vi "configureForCurrentOutput.vi"(8 "error in (no error)":errorcluster, 11 "AnalogOutput in":refnum<class "AnalogOutput.lvclass">) -> (0 "error out":errorcluster, 3 "AnalogOutput out":refnum<class "AnalogOutput.lvclass">)   [LabVIEW 2011, in "Hardware.lvlib" / "Channels.lvlib" / "AnalogOutput.lvclass"]
uses:
  AnalogOutput.lvclass
panel:
  in  "Output Properties":T1
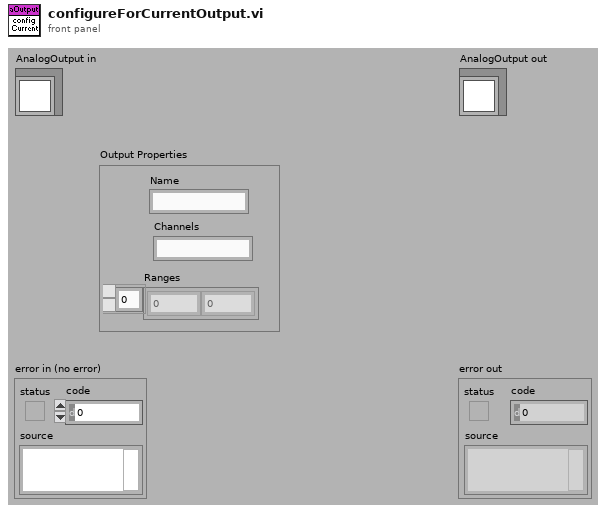
[diagram p1: front panel]
types:
  T1 = cluster{"Name":string, "Channels":string, "Ranges":dbl[]}
  T2 = cluster{"Configuration Type":cluster{"Differential":i16, "Pseudodifferential":i16, "RSE":dbl}, "Output Type":cluster{"Voltage":string, "Current":string, "Standard Function ":cluster{"Sine":string, "Square":string, "Triangle":string}}}
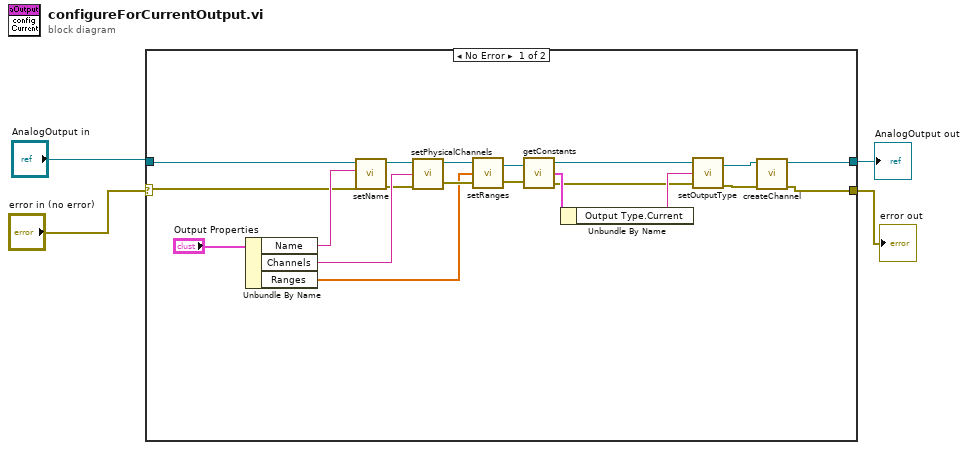
[diagram p0: block diagram]
diagram:
  n1 = case shown="No Error" "error in (no error)" {
    selector: "error in (no error)" -> [w8 w26]
    tunnel: [w7 w26] -> w3
    tunnel: [w6 w25] -> w1
    tunnel: "AnalogOutput in" -> [w9 w25]
    frame No Error {
      n2 = Unbundle By Name("Output Properties") -> ("Name"=w23:string, "Channels"=w21:string, "Ranges"=w5:dbl[])
      n3 = call "setName.vi"("error in (no error)"=w8, "name"=w23, "AnalogOutput.lvclass in"=w9) -> ("error out"=w20:errorcluster, "AnalogOutput.lvclass out"=w22:refnum<class "AnalogOutput.lvclass">)  [unwired: 7 in]
      n4 = call-dynamic "setPhysicalChannels.vi"("error in (no error)"=w20, "Physical Channels"=w21, "AnalogOutput.lvclass in"=w22) -> ("error out"=w18:errorcluster, "AnalogOutput.lvclass out"=w19:refnum<class "AnalogOutput.lvclass">)
      n5 = call "setRanges.vi"("error in (no error)"=w18, "Ranges"=w5, "AnalogOutput.lvclass in"=w19) -> ("error out"=w16:errorcluster, "AnalogOutput.lvclass out"=w17:refnum<class "AnalogOutput.lvclass">)
      n6 = call-dynamic "getConstants.vi"("AnalogOutput in"=w17, "error in (no error)"=w16) -> ("AnalogOutput out"=w13:refnum<class "AnalogOutput.lvclass">, "Constants"=w15:T2, "error out"=w12:errorcluster)
      n7 = Unbundle By Name(w15) -> ("Output Type.Current"=w14:string)
      n8 = call "setOutputType.vi"("error in (no error)"=w12, "Output Type"=w14, "AnalogOutput in"=w13) -> ("error out"=w10:errorcluster, "AnalogOutput out"=w11:refnum<class "AnalogOutput.lvclass">)
      n9 = call-dynamic "createChannel.vi"("error in (no error)"=w10, "AnalogOutput in"=w11) -> ("error out"=w7:errorcluster, "AnalogOutput out"=w6:refnum<class "AnalogOutput.lvclass">)  [unwired: 8 in]
    }
    frame Error {
    }
  }
  "error out" <- w3
  "AnalogOutput out" <- w1
